vi "gfitsio-get-image-type.vi"(8 "error in (no error)":errorcluster, 11 "gfits refnum":T2) -> (0 "error out":errorcluster, 1 "cfitsio datatype":T1 items=["TBIT"=1, "TBYTE  (U8)"=11, "TSBYTE  (I8)"=12, "TLOGICAL"=14, "TSTRING"=16, "TUSHORT  (U16)"=20, "TSHORT  (I16)"=21, "TUINT"=31, "TULONG  (U32)"=40, "TLONG  (I32)"=41, "TFLOAT  (SGL)"=42, "TLONGLONG  (I64)"=81, "TDOUBLE  (DBL)"=82, "TCOMPLEX  (CSG)"=83, "TDOUBLECOMPLEX  (CDB)"=163], 2 "bitpix":T3 items=["<invalid type>"=0, "BYTE_IMG  (U8)"=8, "SHORT_IMG  (I16)"=16, "USHORT_IMG  (U16)"=20, "LONG_IMG  (I32)"=32, "ULONG_IMG  (U32)"=40, "FLOAT_IMG  (SGL)"=-32, "DOUBLE_IMG  (DBL)"=-64], 3 "dup gfits refnum":T2)   [LabVIEW 2014, in "gfitsio.lvlib"]
doc: "Get the equivalent data type of the image. If the image pixel values are scaled, with non-default values for the BZERO and BSCALE keywords, then the routine will return the 'equivalent' data type that is needed to store the scaled values. For example, if BITPIX = 16 and BSCALE = 0.1 then the equivalent data type is FLOAT_IMG. Similarly if BITPIX = 16, BSCALE = 1, and BZERO = 32768, then the the pixel values span the range of an unsigned short integer and the returned data type will be USHORT_IMG. Otherwise the physical data type of the FITS image, as given by the BITPIX keyword, is returned."
uses:
  gfitsio.lvlib
  cfitsio-bitpix.ctl
  gfitsio-refnum.ctl
  cfitsio-datatypes.ctl
  gfitsio.dll
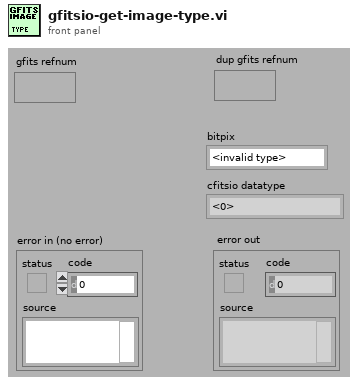
[diagram p1: front panel]
types:
  T1 = typedef "gfitsio.lvlib/cfitsio-datatypes.ctl" = i32
  T2 = typedef "gfitsio.lvlib/gfitsio-refnum.ctl" = refnum<k1>
  T3 = typedef "gfitsio.lvlib/cfitsio-bitpix.ctl" = i32
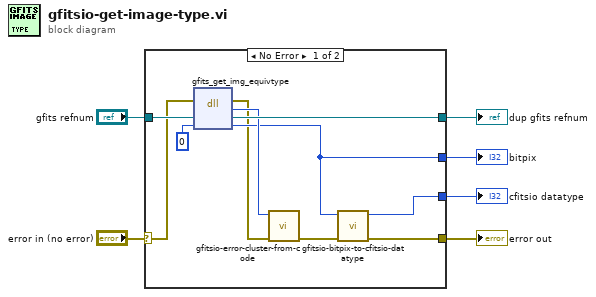
[diagram p0: block diagram]
diagram:
  n1 = case shown="No Error" "error in (no error)" {
    selector: "error in (no error)" -> [w8 w17]
    tunnel: "gfits refnum" -> [w16 w18]
    tunnel: [w10 _] -> w5
    tunnel: [w15 w18] -> w4
    tunnel: [w11 w17] -> w3
    tunnel: [w9 _] -> w1
    frame No Error {
      n2 = dll-call lib="D:/optics_and_proj_related_stuff/labview_codes/gfitsio/gfitsio.dll" fn="gfits_get_img_equivtype"(error in=w8, "handle"=w16, "bitpix"=0) -> (error out=w7:errorcluster, "return type"=w14:i32, "handle"=w15:T2, "bitpix"=w10:i32)  [unwired: 2 in, 1 out]
      n3 = call "gfitsio-error-cluster-from-code.vi"("error in (no error)"=w7, "error code"=w14) -> ("error out"=w12:errorcluster)  [unwired: 9 in]
      n4 = call "gfitsio-bitpix-to-cfitsio-datatype.vi"("error in (no error)"=w12, "bitpix"=w10) -> ("error out"=w11:errorcluster, "cfitsio datatype"=w9:T1)  [unwired: 8 in]
    }
    frame Error {
    }
  }
  "bitpix" <- w5
  "dup gfits refnum" <- w4
  "error out" <- w3
  "cfitsio datatype" <- w1
